vi "speed_to_angle.vi"(1 "Counter Direction":T1, 2 "Counter Value":i32) -> (0 "Output":dbl)   [LabVIEW 2021, in "System.lvclass"]
uses:
  System.lvclass
  <vilib>/myRIO/Common/Instrument Driver Framework/myRIO v1.0/Encoder/typedefs/Encoder Count Direction Enum.ctl
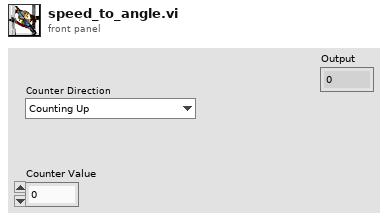
[diagram p1: front panel]
types:
  T1 = typedef "Encoder Count Direction Enum.ctl" = enum16{"Counting Up", "Counting Down"}
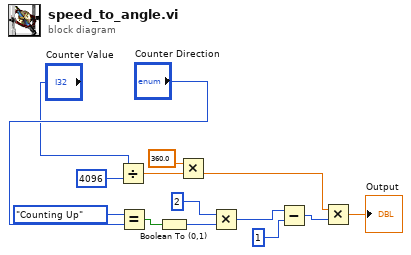
[diagram p0: block diagram]
diagram:
  n1 = Divide(x="Counter Value", y=4096) -> (x/y=w12:dbl)
  n2 = Equal?(x=Encoder_Count_Direction_Enum."Counting Up", y="Counter Direction") -> (x = y?=w8:bool)
  n3 = Boolean To (0,1)(Boolean=w8) -> (0, 1=w9:i16)
  n4 = Multiply(x=360.0, y=w12) -> (x*y=w13:dbl)
  n5 = Multiply(x=i16 2, y=w9) -> (x*y=w2:i16)
  n6 = Subtract(x=w2, y=i16 1 ("x")) -> (x-y=w11:i16)
  n7 = Multiply(x=w13, y=w11) -> (x*y=→"Output":dbl)
